vi "Configure Calibration.vi"(0 "VISA resource name":refnum<visa-resource-name>, 1 "Port 1 (1)":i32=1, 2 "Port 2 (1)":i32=1, 3 "Port 3 (1)":i32=1, 5 "error in (no error)":errorcluster, 6 "Channel (1)":i32=1, 7 "Error Correction State (F: Disable)":bool, 8 "Cal Kit (1)":i32=1, 9 "Velocity Factor (1.0)":dbl=1.0 format="%.2f", 10 "Calibration Type (6: Full 4-port)":u16(ring)=6 items=["Open", "Short", "Through", "1-port", "Full 2-port", "Full 3-port", "Full 4-port", "Enhanced Response", "Gain Phase Open", "Gain Phase Short", "Gain Phase Through", "Gain Phase 1 port "], 11 "Calibration Property Display (F: Disable)":bool, 13 "z0 (50.0)":dbl=50.0 format="%.3f") -> (14 "VISA resource name out":refnum<visa-resource-name>, 19 "error out":errorcluster)   [LabVIEW 2018, in "Agilent ENA Series.lvlib"]
doc: "Configures the calibration parameters.\n\n<b>Note:</b>\nThis VI is not supported by the E5063A or E5080A."
uses:
  Agilent ENA Series.lvlib
panel:
  # "Note:\nThis VI is not supported by the E5063A or E5080A."
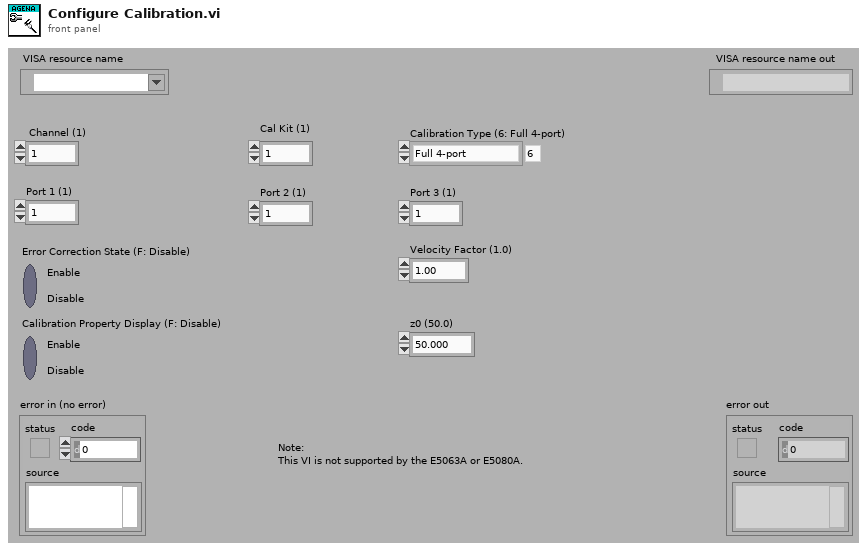
[diagram p1: front panel]
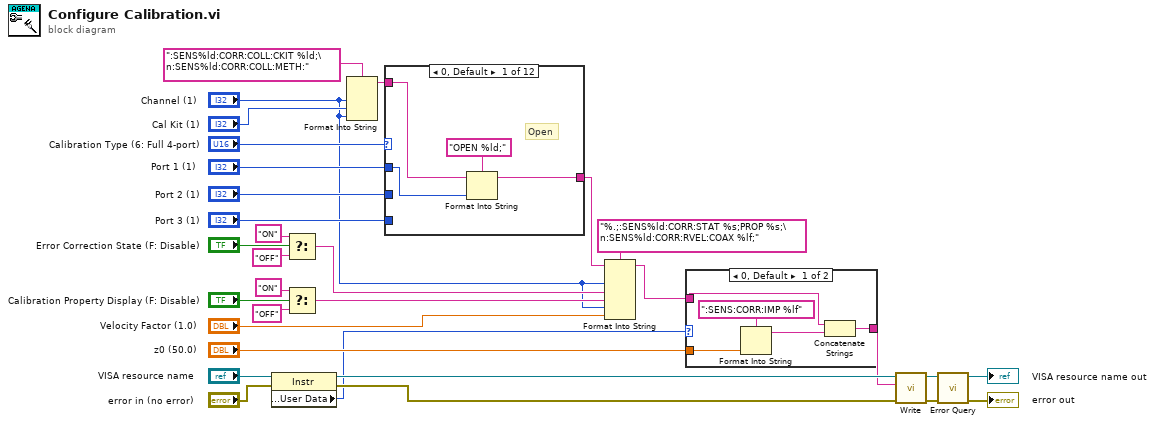
[diagram p0: block diagram]
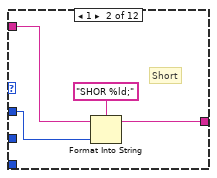
[diagram p3: hidden frame]
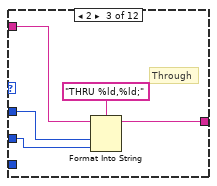
[diagram p4: hidden frame]
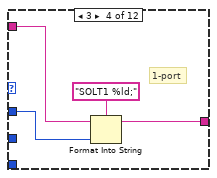
[diagram p5: hidden frame]
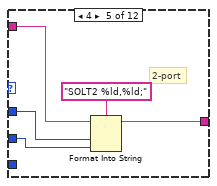
[diagram p6: hidden frame]
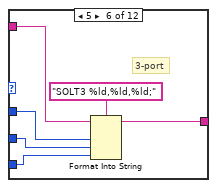
[diagram p7: hidden frame]
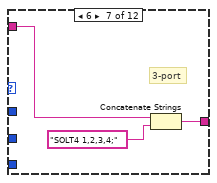
[diagram p8: hidden frame]
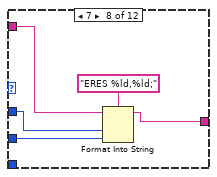
[diagram p9: hidden frame]
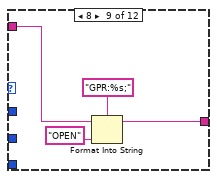
[diagram p10: hidden frame]
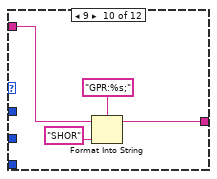
[diagram p11: hidden frame]
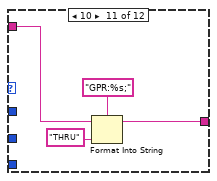
[diagram p12: hidden frame]
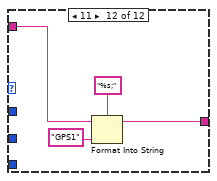
[diagram p13: hidden frame]
diagram:
  n1 = property class="Instr"(reference="VISA resource name", error in="error in (no error)") -> (reference out=w7:refnum<visa-resource-name>, error out=w6:errorcluster, "General Settings:User Data"=w4:u32)
  n2 = Select(t="ON", s="Error Correction State (F: Disable)", f="OFF") -> (s? t:f=w20:string)
  n3 = Select(t="ON", s="Calibration Property Display (F: Disable)", f="OFF") -> (s? t:f=w16:string)
  n4 = Format Into String(format string=":SENS%ld:CORR:COLL:CKIT %ld;\n:SENS%ld:CORR:COLL:METH:", "Channel (1)", "Cal Kit (1)", "Channel (1)") -> (resulting string=w27:string)  [unwired: 2 in, 1 out]
  n5 = case shown="0, Default" "Calibration Type (6: Full 4-port)" {
    tunnel: "Port 1 (1)" -> [w34 w38 w43 w47 w52 w58 _ w65 _ _ _ _]
    tunnel: w27 -> [w33 w37 w42 w46 w51 w57 w62 w66 w69 w73 w77 w81]
    tunnel: [w32 w36 w41 w45 w50 w56 w60 w63 w68 w72 w76 w80] -> w2
    tunnel: "Port 2 (1)" -> [_ _ w40 _ w49 w55 _ w64 _ _ _ _]
    tunnel: "Port 3 (1)" -> [_ _ _ _ _ w54 _ _ _ _ _ _]
    frame 0, Default {
      # "Open"
      n6 = Format Into String(format string="OPEN %ld;", initial string=w33, w34) -> (resulting string=w32:string)  [unwired: 1 in, 1 out]
    }
    frame 1 {
      # "Short"
      n7 = Format Into String(format string="SHOR %ld;", initial string=w37, w38) -> (resulting string=w36:string)  [unwired: 1 in, 1 out]
    }
    frame 2 {
      # "Through"
      n8 = Format Into String(format string="THRU %ld,%ld;", initial string=w42, w43, w40) -> (resulting string=w41:string)  [unwired: 1 in, 1 out]
    }
    frame 3 {
      # "1-port"
      n9 = Format Into String(format string="SOLT1 %ld;", initial string=w46, w47) -> (resulting string=w45:string)  [unwired: 1 in, 1 out]
    }
    frame 4 {
      # "2-port"
      n10 = Format Into String(format string="SOLT2 %ld,%ld;", initial string=w51, w52, w49) -> (resulting string=w50:string)  [unwired: 1 in, 1 out]
    }
    frame 5 {
      # "3-port"
      n11 = Format Into String(format string="SOLT3 %ld,%ld,%ld;", initial string=w57, w58, w55, w54) -> (resulting string=w56:string)  [unwired: 1 in, 1 out]
    }
    frame 6 {
      # "3-port"
      n12 = Concatenate Strings(w62, "SOLT4 1,2,3,4;" ("format string")) -> (w60:string)
    }
    frame 7 {
      n13 = Format Into String(format string="ERES %ld,%ld;", initial string=w66, w65, w64) -> (resulting string=w63:string)  [unwired: 1 in, 1 out]
    }
    frame 8 {
      n14 = Format Into String(format string="GPR:%s;", initial string=w69, "OPEN" ("input 1")) -> (resulting string=w68:string)  [unwired: 1 in, 1 out]
    }
    frame 9 {
      n15 = Format Into String(format string="GPR:%s;", initial string=w73, "SHOR" ("input 1")) -> (resulting string=w72:string)  [unwired: 1 in, 1 out]
    }
    frame 10 {
      n16 = Format Into String(format string="GPR:%s;", initial string=w77, "THRU" ("input 1")) -> (resulting string=w76:string)  [unwired: 1 in, 1 out]
    }
    frame 11 {
      n17 = Format Into String(format string="%s;", initial string=w81, "GPS1" ("input 1")) -> (resulting string=w80:string)  [unwired: 1 in, 1 out]
    }
  }
  n18 = Format Into String(format string="%.;:SENS%ld:CORR:STAT %s;PROP %s;\n:SENS%ld:CORR:RVEL:COAX %lf;", initial string=w2, "Channel (1)", w20, w16, "Channel (1)", "Velocity Factor (1.0)") -> (resulting string=w3:string)  [unwired: 1 in, 1 out]
  n19 = case shown="0, Default" w4 {
    tunnel: "z0 (50.0)" -> [w87 _]
    tunnel: w3 -> [w85 w89]
    tunnel: [w84 w89] -> w1
    frame 0, Default {
      n20 = Format Into String(format string=":SENS:CORR:IMP %lf", w87) -> (resulting string=w86:string)  [unwired: 2 in, 1 out]
      n21 = Concatenate Strings(w85, w86) -> (w84:string)
    }
    frame 2..4 {
    }
  }
  n22 = call "Write.vi"("error in (no error)"=w6, "String ()"=w1, "VISA resource name"=w7) -> ("error out"=w12:errorcluster, "VISA resource name out"=w13:refnum<visa-resource-name>)  [unwired: 6 in, 1 out]
  n23 = call "Error Query.vi"("error in (no error)"=w12, "VISA resource name"=w13) -> ("error out"=→"error out":errorcluster, "VISA resource name out"=→"VISA resource name out":refnum<visa-resource-name>)  [unwired: 6 in, 2 out]
